vi "Get Ingredients.vi"(8 "error in (no error)":errorcluster, 11 "Battery Stack in":refnum<class "Battery Stack.lvclass">) -> (0 "error out":errorcluster, 2 "Ingredients":T1[](array[typedef]), 3 "Battery Stack out":refnum<class "Battery Stack.lvclass">)   [LabVIEW 2020, in "Battery Stack.lvclass"]
uses:
  Battery Stack.lvclass
  Item/Ingredient.ctl
  Item/Item.lvclass
  Chemicals/Chemicals.lvclass
  C:/dev/IlluminatedG/lv-oopanel-gc-calc/Item/Item.lvclass
  Metal/Metal.lvclass
  Plastic/Plastic.lvclass
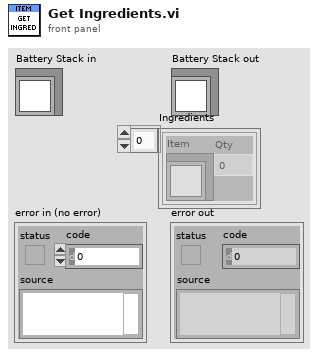
[diagram p1: front panel]
types:
  T1 = typedef "Item.lvclass/Ingredient.ctl" = cluster{"Item":refnum<class "Item.lvclass">, "Qty":dbl}
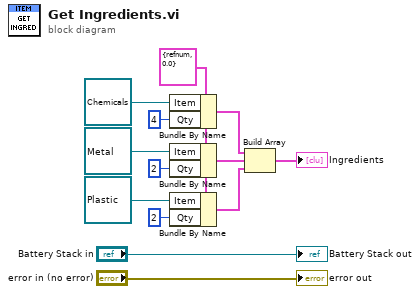
[diagram p0: block diagram]
diagram:
  w5 = T1 {"Item"=refnum, "Qty"=0.0} ("Ingredient")
  n1 = Bundle By Name(cluster=w5, "Item"=refnum<class "Chemicals.lvclass"> refnum ("Chemicals.lvclass"), "Qty"=4) -> (w2:T1)
  n2 = Bundle By Name(cluster=w5, "Item"=refnum<class "Metal.lvclass"> refnum ("Metal.lvclass"), "Qty"=2) -> (w4:T1)
  n3 = Bundle By Name(cluster=w5, "Item"=refnum<class "Plastic.lvclass"> refnum ("Plastic.lvclass"), "Qty"=2) -> (w3:T1)
  n4 = Build Array(w2, w4, w3) -> (→"Ingredients":T1[])
  "error out" <- "error in (no error)"
  "Battery Stack out" <- "Battery Stack in"
